vi "Test Remote Client - Copy.vi"(9 "Array size":i32=10000, 10 "Number of Messages":i32=200) -> (0 "<time/message (ms)>":i32, 1 "bytes/second":dbl, 2 "messages/second":dbl, 3 "<size>":i32)   [LabVIEW 2016]
uses:
  lvsrc/SMOs/RemoteControl.STM/RemoteControl.STM.lvclass
  C:/user/patrick/hg/levylab_inst/lvsrc/SMOs/RemoteControl/RemoteControl.lvclass
  lvsrc/SMOs/RemoteControl/RemoteControl.lvclass
panel:
  out "length":i32=80004
  in  "stop":bool
  out "error out":errorcluster
  out "Data out":variant
  out "Command out":string
  in  "Command":string="HELP"
  in  "address":string
  in  "Port":u16=6341
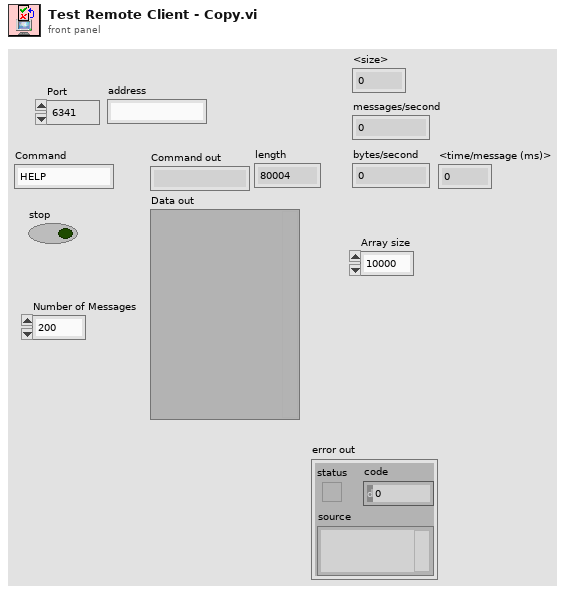
[diagram p1: front panel]
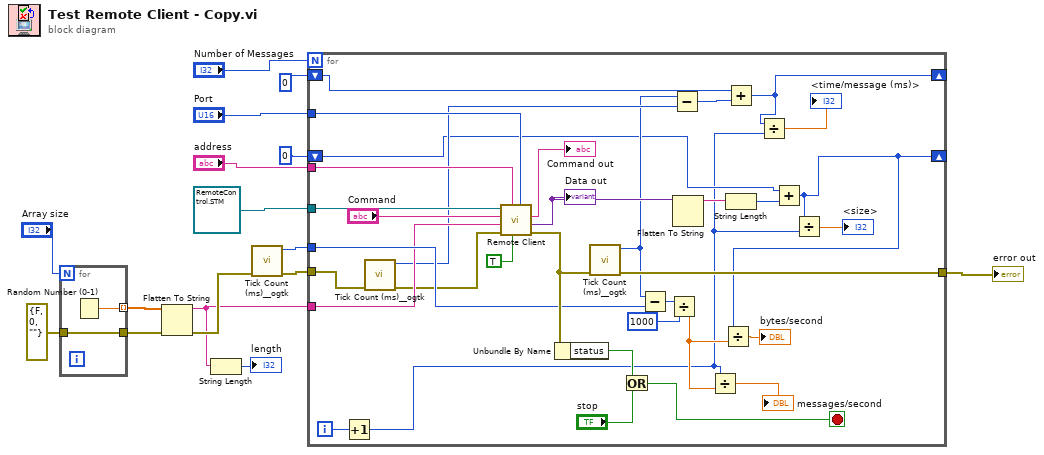
[diagram p0: block diagram]
diagram:
  n1 = for {
    N: "Array size" -> [_]
    tunnel: [w18] -> w7
    tunnel: errorcluster {"status"=FALSE, "code"=0, "source"=""} ("error in (no error)") -> [w18]
    tunnel: [w17] -> w8 mode=indexing
    n2 = Random Number (0-1)() -> (number: 0 to 1=w17:dbl)
  }
  n3 = Flatten To String(anything=w8, error in (no error)=w7) -> (data string=w4:string, error out=w6:errorcluster)  [unwired: 2 in, 1 out]
  n4 = String Length(string=w4) -> (length=→"length":i32)
  n5 = call <userlib>:"Tick Count (ms)__ogtk.vi"("error in (no error)"=w6) -> ("error out"=w12:errorcluster, "millisecond timer value"=w11:u32)  [unwired: 9 in]
  n6 = for {
    N: "Number of Messages" -> [_]
    tunnel: refnum<class "RemoteControl.STM.lvclass"> refnum ("RemoteControl.STM.lvclass") -> [w52]
    tunnel: "Port" -> [w51]
    tunnel: [w46] -> w13
    tunnel: "address" -> [w50]
    tunnel: w12 -> [w30]
    tunnel: w11 -> [w41]
    tunnel: w4 -> [w33]
    shift-right: [w21] -> _
    shift-left: 0 -> [w24]
    shift-right: [w22] -> _
    shift-left: 0 -> [w23]
    i -> [w42]
    stop <- w32 stop-if-true
    n7 = Increment(x=w42) -> (x+1=w20:i32)
    n8 = call <userlib>:"Tick Count (ms)__ogtk.vi"("error in (no error)"=w30) -> ("error out"=w29:errorcluster, "millisecond timer value"=w28:u32)  [unwired: 9 in]
    n9 = call "Remote Client.vi"("Port"=w51, "Wait for Response?"=TRUE, "address"=w50, "error in (no error)"=w29, "Data"=w33, "Command"="Command", "RemoteControl in"=w52) -> ("error out"=w45:errorcluster, "Data out"=w37:variant, "Command out"=→"Command out":string)  [unwired: 1 in, 1 out]
    "Data out" <- w37
    n10 = Unbundle By Name(w45) -> ("status"=w43:bool)
    n11 = call <userlib>:"Tick Count (ms)__ogtk.vi"("error in (no error)"=w45) -> ("error out"=w46:errorcluster, "millisecond timer value"=w27:u32)  [unwired: 9 in]
    n12 = Or(x=w43, y="stop") -> (x .or. y?=w32:bool)
    n13 = Subtract(x=w27, y=w41) -> (x-y=w40:u32)
    n14 = Divide(x=w40, y=u32 1000) -> (x/y=w35:dbl)
    n15 = Subtract(x=w27, y=w28) -> (x-y=w26:u32)
    n16 = Flatten To String(anything=w37) -> (data string=w36:string)  [unwired: 3 in, 2 out]
    n17 = Divide(x=w20, y=w35) -> (x/y=→"messages/second":dbl)
    n18 = Add(x=w23, y=w26) -> (x+y=w22:u32)
    n19 = String Length(string=w36) -> (length=w31:i32)
    n20 = Divide(x=w22, y=w20) -> (x/y=→"<time/message (ms)>":dbl)
    n21 = Add(x=w24, y=w31) -> (x+y=w21:i32)
    n22 = Divide(x=w21, y=w35) -> (x/y=→"bytes/second":dbl)
    n23 = Divide(x=w21, y=w20) -> (x/y=→"<size>":dbl)
  }
  "error out" <- w13
